vi "Insert Drop Shadow.vi"(6 "Variant in":variant, 7 "Shift Pressed?":bool, 8 "error in (no error)":errorcluster, 10 "QD Combo Box Ref":refnum<vi>, 11 "QD Launch VI Ref":refnum<vi>) -> (0 "error out":errorcluster, 4 "Variant out":variant)   [LabVIEW 2019]
doc: "Add drop shadows to a decoration(s) on the front panel.\n\nDefault Shortcut - [S]"
uses:
  <vilib>/Utility/miscctls.llb/LVPositionTypeDef.ctl
  d952363f-c180-47b2-840b-fbb039c5fedd.vi
panel:
  in  "Undo Name":string="Insert Drop Shadow"
  # "Do not change the connector pane of this VI.\n\nSee the block diagram for directions on how to use this template."
  # "Specify the name of the Undo transaction"
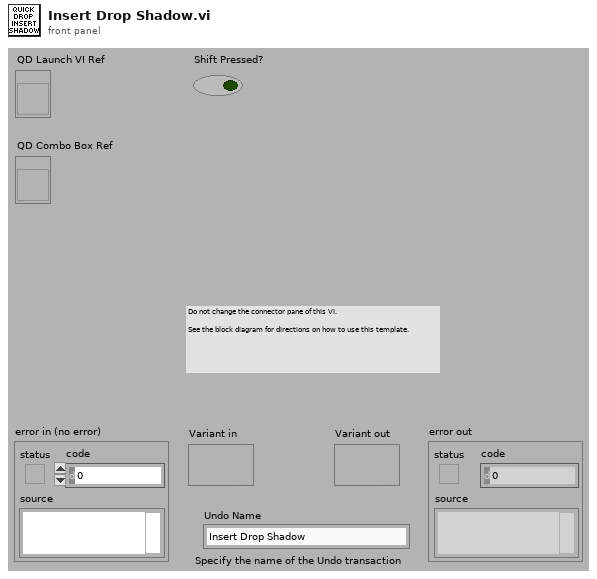
[diagram p1: front panel]
types:
  T1 = typedef "LVPositionTypeDef.ctl" = cluster{"Left":i32, "Top":i32}
  T2 = typedef "LVRectTypeDef.ctl" = cluster{"Left":i16, "Top":i16, "Right":i16, "Bottom":i16}
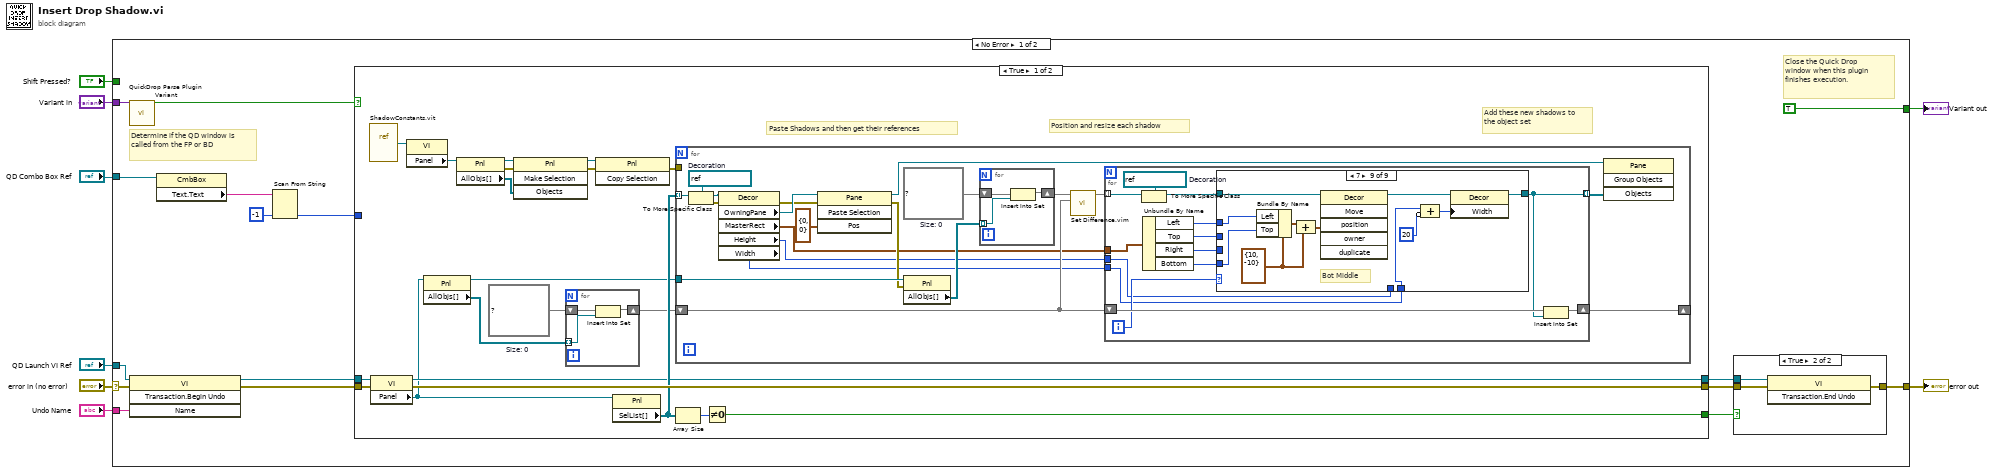
[diagram p0: block diagram]
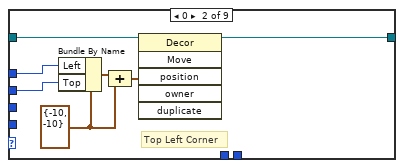
[diagram p3: hidden frame]
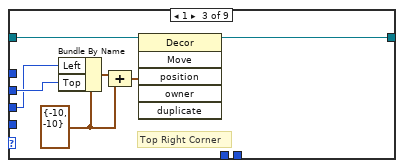
[diagram p4: hidden frame]
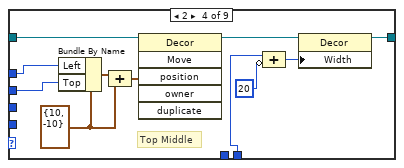
[diagram p5: hidden frame]
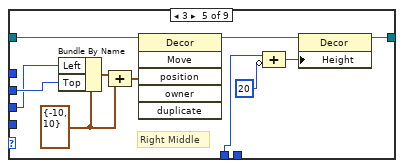
[diagram p6: hidden frame]
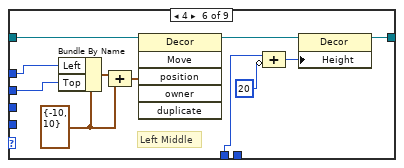
[diagram p7: hidden frame]
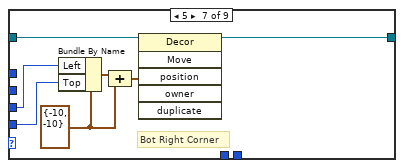
[diagram p8: hidden frame]
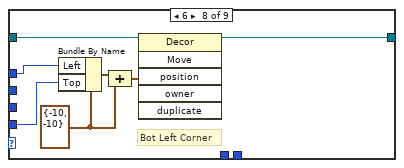
[diagram p9: hidden frame]
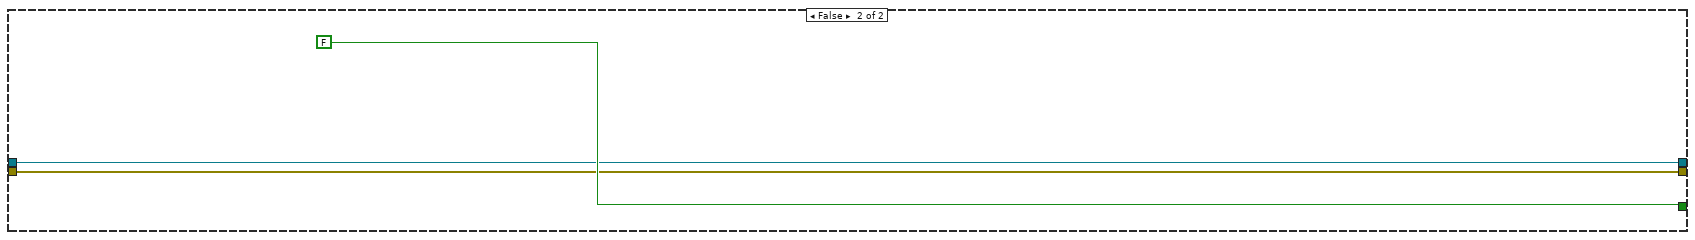
[diagram p10: hidden frame]
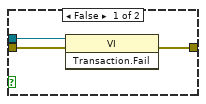
[diagram p11: hidden frame]
diagram:
  n1 = case shown="No Error" "error in (no error)" {
    selector: "error in (no error)" -> [w23 w167]
    tunnel: [w17 w167] -> w7
    tunnel: "QD Launch VI Ref" -> [w22 _]
    tunnel: "Shift Pressed?" -> [_ _]
    tunnel: "QD Combo Box Ref" -> [w15 _]
    tunnel: "Variant in" -> [w24 _]
    tunnel: "Undo Name" -> [w21 _]
    tunnel: [TRUE _] -> w1
    frame No Error {
      # "Close the Quick Drop window when this plugin finishes execution."
      # "Determine if the QD window is called from the FP or BD"
      n2 = call <vilib>:"QuickDrop Parse Plugin Variant.vi"("QDKS Variant in"=w24) -> ("QD Launch VI Panel?"=w19:bool)  [unwired: 12 in, 2 out]
      n3 = invoke class="VI" method="Transaction.Begin Undo"(reference=w22, error in=w23, "Name"=w21) -> (reference out=w16:refnum<vi>, error out=w18:errorcluster)  [unwired: 1 in, 2 out]
      n4 = property class="CmbBox"(reference=w15) -> ("Text.Text"=w14:string)  [unwired: 1 in, 2 out]
      n5 = Scan From String(input string=w14, default 1=-1 ("Max Rows (-1)")) -> (output 1=w12:i32)  [unwired: 3 in, 3 out]
      n6 = case shown="True" w19 {
        tunnel: w18 -> [w43 w158]
        tunnel: w16 -> [w44 w159]
        tunnel: w12 -> [_ _]
        tunnel: [w30 w159] -> w11
        tunnel: [w42 w158] -> w10
        tunnel: [w40 FALSE] -> w9
        frame True {
          w27 = set{refnum<vi>} {}  # Size: 0
          # "Paste Shadows and then get their references"
          # "Position and resize each shadow"
          # "Add these new shadows to the object set"
          n7 = vi-ref "ShadowConstants.vit"() -> (w38:refnum<vi>)
          n8 = property class="VI"(reference=w44, error in=w43) -> (reference out=w30:refnum<vi>, error out=w42:errorcluster, "Panel"=w29:refnum<vi>)
          n9 = property class="VI"(reference=w38) -> ("Panel"=w32:refnum<vi>)  [unwired: 1 in, 2 out]
          n10 = property class="Pnl"(reference=w29) -> (reference out=w28:refnum<vi>, "AllObjs[]"=w26:refnum<vi>[])  [unwired: 1 in, 1 out]
          n11 = property class="Pnl"(reference=w32) -> (reference out=w33:refnum<vi>, error out=w34:errorcluster, "AllObjs[]"=w35:refnum<vi>[])  [unwired: 1 in]
          n12 = invoke class="Pnl" method="Make Selection"(reference=w33, error in=w34, "Objects"=w35) -> (reference out=w36:refnum<vi>, error out=w37:errorcluster)  [unwired: 1 in, 2 out]
          n13 = for {
            tunnel: w26 -> [w47] mode=indexing
            shift-right: [w45] -> w25
            shift-left: w27 -> [w46]
            n14 = Insert Into Set(10:w47, 11:w46) -> (3:w45:set{refnum<vi>})  [unwired: 1 out]
          }
          n15 = invoke class="Pnl" method="Copy Selection"(reference=w36, error in=w37) -> (error out=w31:errorcluster)  [unwired: 1 in, 2 out]
          n16 = property class="Pnl"(reference=w29) -> ("SelList[]"=w39:refnum<vi>[])  [unwired: 1 in, 2 out]
          n17 = for {
            tunnel: w39 -> [w64] mode=indexing
            tunnel: w31 -> [_]
            tunnel: w28 -> [w61]
            shift-right: [w54] -> _
            shift-left: w25 -> [w55]
            w60 = set{refnum<vi>} {}  # Size: 0
            w67 = refnum<vi> refnum  # Decoration
            n18 = To More Specific Class(target class=w67, reference=w64) -> (specific class reference=w66:refnum<vi>, error out=w65:errorcluster)  [unwired: 1 in]
            n19 = property class="Decor"(reference=w66, error in=w65) -> (error out=w62:errorcluster, "OwningPane"=w63:refnum<vi>, "MasterRect"=w52:T2, "Height"=w51:u32, "Width"=w50:u32)  [unwired: 1 out]
            n20 = invoke class="Pane" method="Paste Selection"(reference=w63, error in=w62, "Pos"=T1 {"Left"=0, "Top"=0} ("Position")) -> (reference out=w49:refnum<vi>, error out=w59:errorcluster)  [unwired: 1 in, 2 out]
            n21 = property class="Pnl"(reference=w61, error in=w59) -> ("AllObjs[]"=w58:refnum<vi>[])  [unwired: 2 out]
            n22 = for {
              tunnel: w58 -> [w157] mode=indexing
              shift-right: [w155] -> w57
              shift-left: w60 -> [w156]
              n23 = Insert Into Set(10:w157, 11:w156) -> (3:w155:set{refnum<vi>})  [unwired: 1 out]
            }
            n24 = call "Set Difference.vim"("set 2"=w55, "set 1"=w57) -> ("difference"=w56:set{refnum<vi>})  [unwired: 9 in]
            n25 = for {
              tunnel: w56 -> [w73] mode=indexing
              shift-right: [w80] -> w54
              shift-left: w55 -> [w81]
              tunnel: w52 -> [w78]
              tunnel: w51 -> [w69]
              tunnel: w50 -> [w70]
              tunnel: [w68] -> w48 mode=indexing
              i -> [w79]
              w71 = refnum<vi> refnum  # Decoration
              n26 = To More Specific Class(target class=w71, reference=w73) -> (specific class reference=w72:refnum<vi>)  [unwired: 1 in, 1 out]
              n27 = Unbundle By Name(w78) -> ("Left"=w77:i16, "Top"=w76:i16, "Right"=w75:i16, "Bottom"=w74:i16)
              n28 = case shown="7" w79 {
                tunnel: w72 -> [w82 w89 w96 w107 w118 w129 w132 w139 w154]
                tunnel: [w82 w88 w95 w100 w112 w123 w133 w140 w149] -> w68
                tunnel: w77 -> [_ w84 _ w101 _ w119 _ w137 w146]
                tunnel: w76 -> [_ w83 w91 w102 w113 w124 _ _ _]
                tunnel: w75 -> [_ _ w90 _ w109 _ w131 _ _]
                tunnel: w74 -> [_ _ _ _ _ _ w130 w138 w144]
                tunnel: w70 -> [_ _ _ w97 _ _ _ _ w145]
                tunnel: w69 -> [_ _ _ _ w108 w120 _ _ _]
                frame Default {
                }
                frame 0 {
                  w85 = T1 {"Left"=-10, "Top"=-10} ("position")
                  # "Top Left Corner"
                  n29 = Bundle By Name(cluster=w85, "Left"=w84, "Top"=w83) -> (w87:T1)
                  n30 = Compound Arithmetic op=ADD(w87, w85) -> (w86:T1)
                  n31 = invoke class="Decor" method="Move"(reference=w89, "position"=w86) -> (reference out=w88:refnum<vi>)  [unwired: 4 in, 5 out]
                }
                frame 1 {
                  w92 = T1 {"Left"=-10, "Top"=-10} ("position")
                  # "Top Right Corner"
                  n32 = Bundle By Name(cluster=w92, "Left"=w90, "Top"=w91) -> (w94:T1)
                  n33 = Compound Arithmetic op=ADD(w94, w92) -> (w93:T1)
                  n34 = invoke class="Decor" method="Move"(reference=w96, "position"=w93) -> (reference out=w95:refnum<vi>)  [unwired: 4 in, 5 out]
                }
                frame 2 {
                  w103 = T1 {"Left"=10, "Top"=-10} ("position")
                  # "Top Middle"
                  n35 = Bundle By Name(cluster=w103, "Left"=w101, "Top"=w102) -> (w105:T1)
                  n36 = Compound Arithmetic op=ADD(w105, w103) -> (w104:T1)
                  n37 = invoke class="Decor" method="Move"(reference=w107, "position"=w104) -> (reference out=w106:refnum<vi>)  [unwired: 4 in, 5 out]
                  n38 = Compound Arithmetic op=ADD(w97, invert u32 20 ("value")) -> (w99:u32)
                  n39 = property class="Decor"(reference=w106, "Width"=w99) -> (reference out=w100:refnum<vi>)  [unwired: 1 in, 1 out]
                }
                frame 3 {
                  w114 = T1 {"Left"=-10, "Top"=10} ("position")
                  # "Right Middle"
                  n40 = Bundle By Name(cluster=w114, "Left"=w109, "Top"=w113) -> (w116:T1)
                  n41 = Compound Arithmetic op=ADD(w116, w114) -> (w115:T1)
                  n42 = invoke class="Decor" method="Move"(reference=w118, "position"=w115) -> (reference out=w117:refnum<vi>)  [unwired: 4 in, 5 out]
                  n43 = Compound Arithmetic op=ADD(w108, invert u32 20 ("value")) -> (w111:u32)
                  n44 = property class="Decor"(reference=w117, "Height"=w111) -> (reference out=w112:refnum<vi>)  [unwired: 1 in, 1 out]
                }
                frame 4 {
                  w125 = T1 {"Left"=-10, "Top"=10} ("position")
                  # "Left Middle"
                  n45 = Bundle By Name(cluster=w125, "Left"=w119, "Top"=w124) -> (w127:T1)
                  n46 = Compound Arithmetic op=ADD(w127, w125) -> (w126:T1)
                  n47 = invoke class="Decor" method="Move"(reference=w129, "position"=w126) -> (reference out=w128:refnum<vi>)  [unwired: 4 in, 5 out]
                  n48 = Compound Arithmetic op=ADD(w120, invert u32 20 ("value")) -> (w122:u32)
                  n49 = property class="Decor"(reference=w128, "Height"=w122) -> (reference out=w123:refnum<vi>)  [unwired: 1 in, 1 out]
                }
                frame 5 {
                  w134 = T1 {"Left"=-10, "Top"=-10} ("position")
                  # "Bot Right Corner"
                  n50 = Bundle By Name(cluster=w134, "Left"=w131, "Top"=w130) -> (w136:T1)
                  n51 = Compound Arithmetic op=ADD(w136, w134) -> (w135:T1)
                  n52 = invoke class="Decor" method="Move"(reference=w132, "position"=w135) -> (reference out=w133:refnum<vi>)  [unwired: 4 in, 5 out]
                }
                frame 6 {
                  w141 = T1 {"Left"=-10, "Top"=-10} ("position")
                  # "Bot Left Corner"
                  n53 = Bundle By Name(cluster=w141, "Left"=w137, "Top"=w138) -> (w143:T1)
                  n54 = Compound Arithmetic op=ADD(w143, w141) -> (w142:T1)
                  n55 = invoke class="Decor" method="Move"(reference=w139, "position"=w142) -> (reference out=w140:refnum<vi>)  [unwired: 4 in, 5 out]
                }
                frame 7 {
                  w150 = T1 {"Left"=10, "Top"=-10} ("position")
                  # "Bot Middle"
                  n56 = Bundle By Name(cluster=w150, "Left"=w146, "Top"=w144) -> (w152:T1)
                  n57 = Compound Arithmetic op=ADD(w152, w150) -> (w151:T1)
                  n58 = invoke class="Decor" method="Move"(reference=w154, "position"=w151) -> (reference out=w153:refnum<vi>)  [unwired: 4 in, 5 out]
                  n59 = Compound Arithmetic op=ADD(w145, invert u32 20 ("value")) -> (w148:u32)
                  n60 = property class="Decor"(reference=w153, "Width"=w148) -> (reference out=w149:refnum<vi>)  [unwired: 1 in, 1 out]
                }
              }
              n61 = Insert Into Set(10:w68, 11:w81) -> (3:w80:set{refnum<vi>})  [unwired: 1 out]
            }
            n62 = invoke class="Pane" method="Group Objects"(reference=w49, "Objects"=w48) -> ()  [unwired: 2 in, 4 out]
          }
          n63 = Array Size(array=w39) -> (size(s)=w41:i32)
          n64 = Not Equal To 0?(x=w41) -> (x != 0?=w40:bool)
        }
        frame False {
        }
      }
      n65 = case shown="True" w9 {
        tunnel: [w161 w166] -> w17
        tunnel: w11 -> [w163 w165]
        tunnel: w10 -> [w162 w164]
        frame False {
          n66 = invoke class="VI" method="Transaction.Fail"(reference=w163, error in=w162) -> (error out=w161:errorcluster)  [unwired: 1 in, 2 out]
        }
        frame True {
          n67 = invoke class="VI" method="Transaction.End Undo"(reference=w165, error in=w164) -> (error out=w166:errorcluster)  [unwired: 1 in, 2 out]
        }
      }
    }
    frame Error {
    }
  }
  "error out" <- w7
  "Variant out" <- w1
